vi "ti2_moveHome.vi"(8 "error in (no error)":errorcluster) -> (0 "error out":errorcluster)   [LabVIEW 2018, in "ti2lv.lvlib"]
uses:
  ti2lv.lvlib
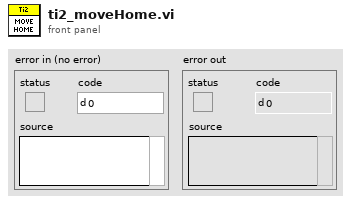
[diagram p1: front panel]
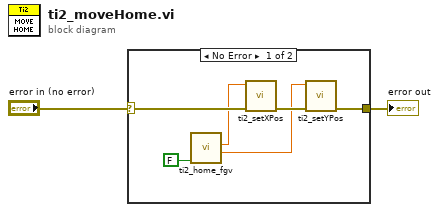
[diagram p0: block diagram]
diagram:
  n1 = case shown="No Error" "error in (no error)" {
    selector: "error in (no error)" -> [w7 w9]
    tunnel: [w6 w9] -> w2
    frame No Error {
      n2 = call "ti2_home_fgv.vi"("Init?"=FALSE) -> ("Y (um) 3"=w3:dbl, "X (um) 2"=w4:dbl)  [unwired: 9 in]
      n3 = call "ti2_setXPos.vi"("error in (no error)"=w7, "x Position (um)"=w4) -> ("error out"=w5:errorcluster)  [unwired: 9 in]
      n4 = call "ti2_setYPos.vi"("error in (no error)"=w5, "y Position (um)"=w3) -> ("error out"=w6:errorcluster)  [unwired: 9 in]
    }
    frame Error {
    }
  }
  "error out" <- w2
